vi "GUI - About.vi"() -> ()   [LabVIEW 2014]
uses:
  Utilities/Global - Demo Mode Flags.vi
panel:
  in  "OK":bool
  in  "Return":bool
  out "About":string
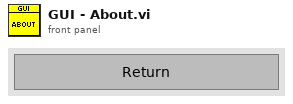
[diagram p1: front panel]
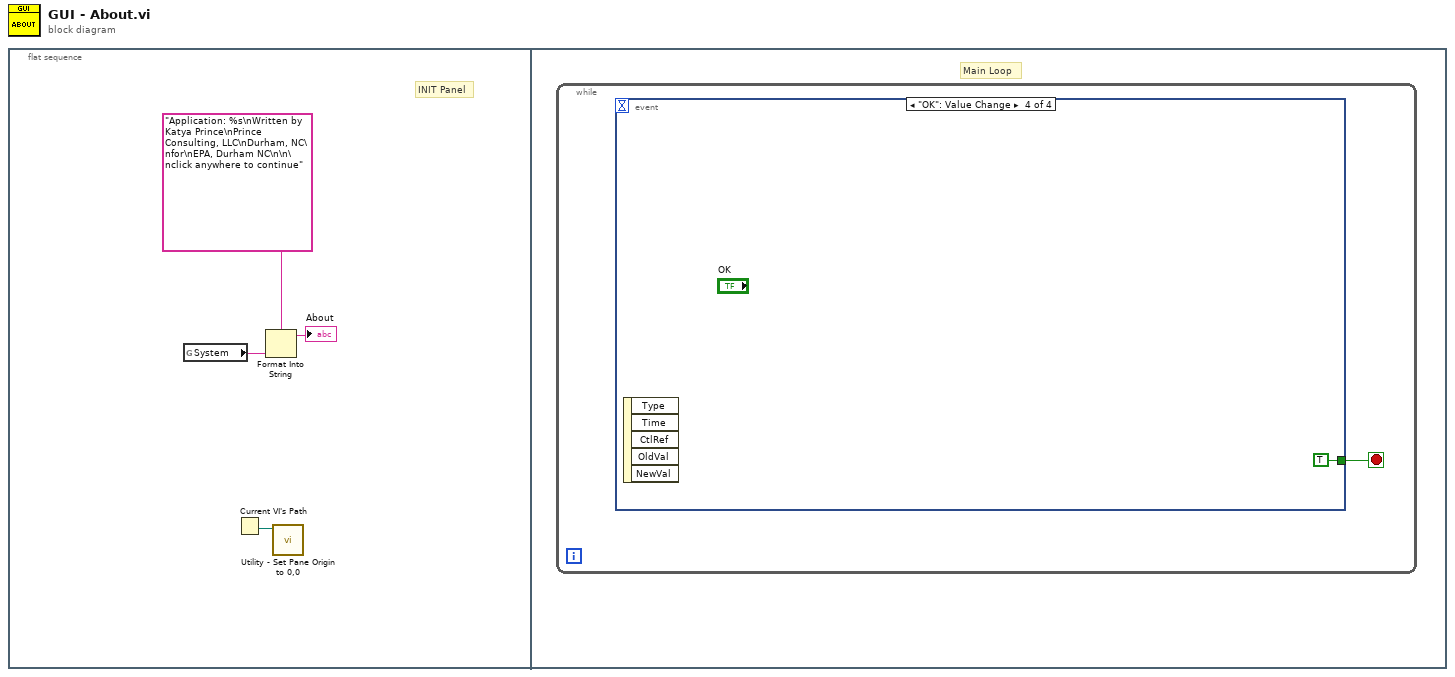
[diagram p0: block diagram]
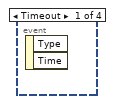
[diagram p2: hidden frame]
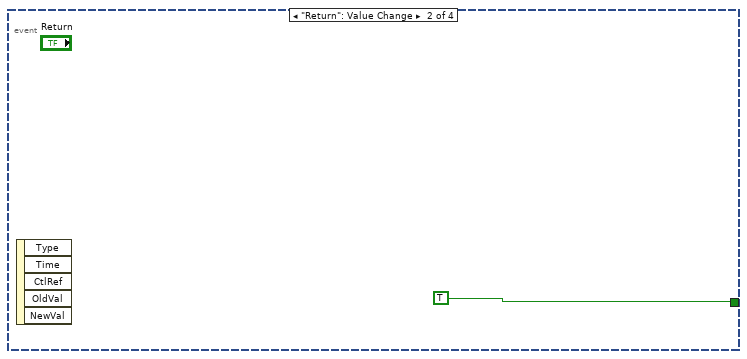
[diagram p3: hidden frame]
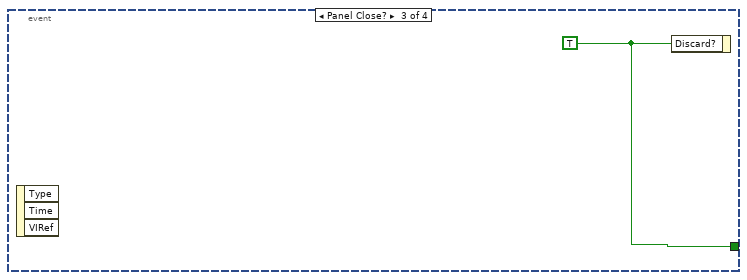
[diagram p4: hidden frame]
diagram:
  n1 = flat-sequence {
    frame #0 {
      # "INIT Panel"
      n2 = global read "Global - Demo Mode Flags.vi" "System"() -> (w3:string)
      n3 = Current VI's Path() -> (path=w4:path)
      n4 = Format Into String(format string="Application: %s\nWritten by Katya Prince\nPrince Consulting, LLC\nDurham, NC\nfor\nEPA, Durham NC\n\n\nclick anywhere to continue", w3) -> (resulting string=→"About":string)  [unwired: 2 in, 1 out]
      n5 = call "Utility - Set Pane Origin to 0,0.vi"("vi path"=w4) -> ()  [unwired: 10 in, 1 out]
    }
    frame #1 {
      # "Main Loop"
      n6 = while {
        stop <- w5 stop-if-true
        n7 = event shown="[3] \"OK\": Value Change" {
          selector: _ -> [_ _ _ _]
          dyn-events: _ -> [_ _ _ _]
          timeout: _ -> [_ _ _ _]
          tunnel: [_ TRUE ("T button?") w7 TRUE ("Discard?")] -> w5
          event Timeout {
            n8 = event-data() -> ()  [unwired: 1 in, 2 out]
          }
          event "Return": Value Change {
            n9 = event-data() -> ()  [unwired: 1 in, 5 out]
          }
          event Panel Close? {
            w7 = TRUE ("Discard?")
            n10 = event-data() -> ()  [unwired: 1 in, 3 out]
            n11 = event-data("Discard?"=w7) -> ()  [unwired: 1 in, 1 out]
          }
          event "OK": Value Change {
            n12 = event-data() -> ()  [unwired: 1 in, 5 out]
          }
        }
      }
    }
  }
